vi "ALTS-2015 LV2GBL Scan trigger Status.vi"(7 "Options":T1=enum."Get", 8 "Error In":errorcluster, 11 "Scan Trigger State in":bool=TRUE) -> (0 "Error Out":errorcluster, 3 "Scan Trigger State Out":bool)   [LabVIEW 2013]
uses:
  Controls/ALTS-2015 LV2GBL Get_Set Option.ctl
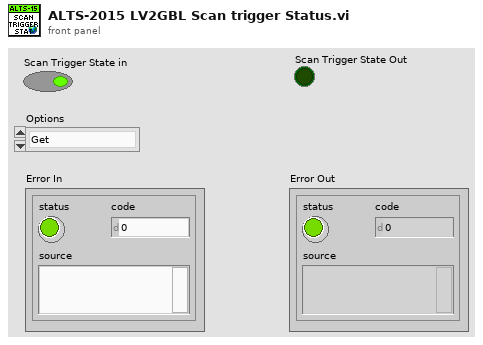
[diagram p1: front panel]
types:
  T1 = typedef "ALTS-2015 LV2GBL Get_Set Option.ctl" = enum16{"Set", "Get"}
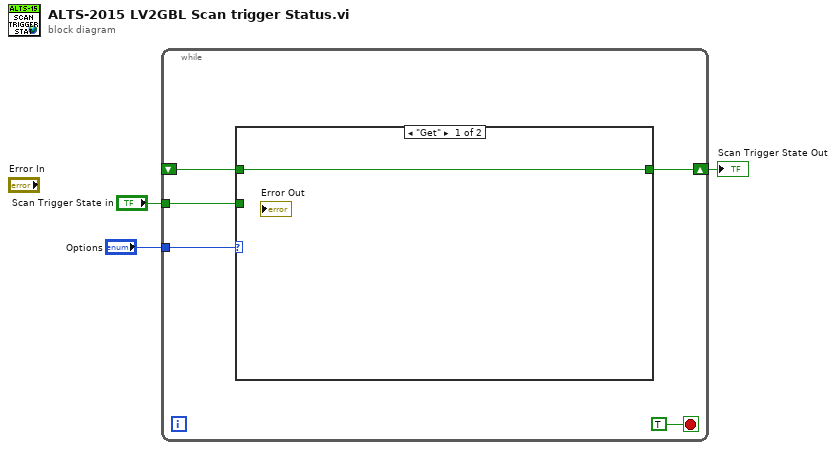
[diagram p0: block diagram]
diagram:
  n1 = while {
    tunnel: "Options" -> [w8]
    tunnel: "Scan Trigger State in" -> [w6]
    shift-right: [w7] -> w1
    shift-left: _ -> [w5]
    stop <- TRUE stop-if-true
    n2 = case shown="\"Get\"" w8 {
      tunnel: [w9 w10] -> w7
      tunnel: w6 -> [_ w10]
      tunnel: w5 -> [w9 _]
      frame "Get" {
      }
      frame "Set" {
      }
    }
  }
  "Scan Trigger State Out" <- w1
